vi "gRPC Client Test.vi"(11 "address":string="localhost:") -> (2 "Loop Counter":i32, 3 "Response Data":T1)   [LabVIEW 2019, in "Generated_client.lvlib"]
uses:
  Generated_client.lvlib
  RPC Messages/helloworld_HelloReply.ctl
panel:
  out "Request cluster":cluster{string}
  in  "stop":bool
  out "response error":errorcluster caption="error out"
  out "no error counter":i32
  out "-1014 error counter":i32
  out "-1004 error counter":i32
  out "-1012 error counter 2":i32
  out "destroy error":errorcluster caption="error out"
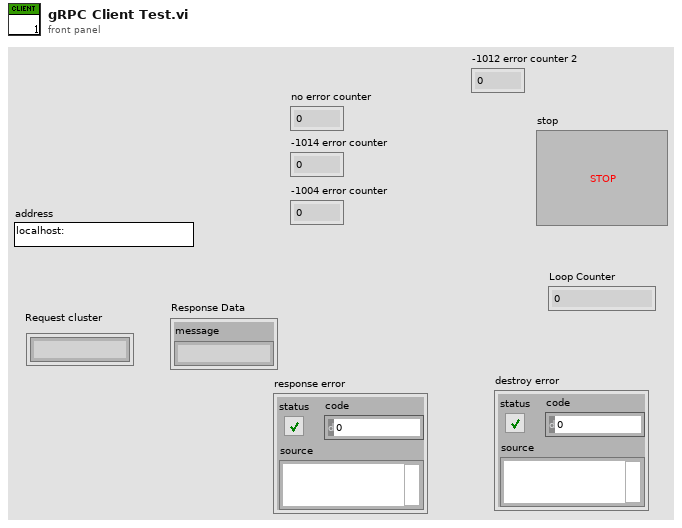
[diagram p1: front panel]
types:
  T1 = typedef "Generated_client.lvlib/helloworld_HelloReply.ctl" = cluster{"message":string}
  T2 = typedef "grpc-lvsupport-release.lvlib/grpcId.ctl" = u64
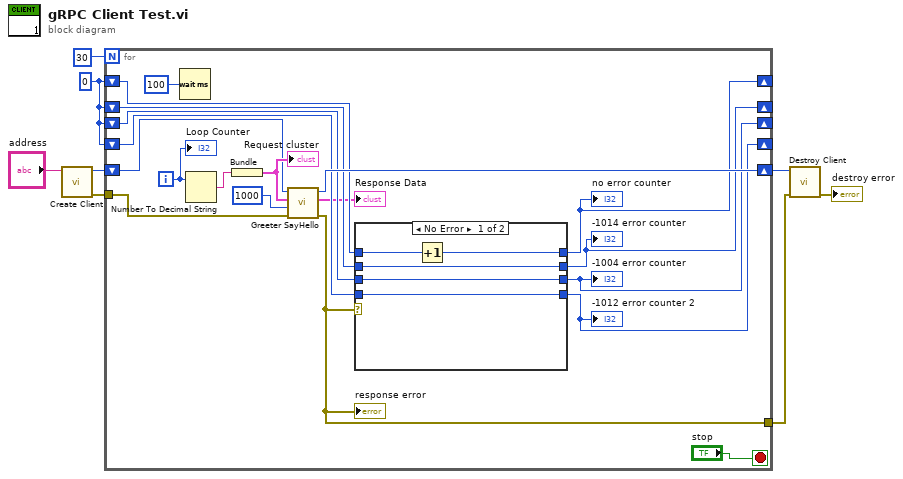
[diagram p0: block diagram]
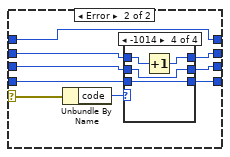
[diagram p2: hidden frame]
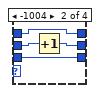
[diagram p4: hidden frame]
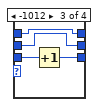
[diagram p5: hidden frame]
diagram:
  w8 = 0
  n1 = call "Create Client.vi"("address"="address") -> ("error out"=w1:errorcluster, "gRPC ID Out"=w6:T2)  [unwired: 9 in]
  n2 = for {
    N: 30 -> [_]
    shift-right: [w27] -> w5
    shift-left: w6 -> [w14]
    shift-right: [w21] -> _
    shift-left: w8 -> [w22]
    shift-right: [w25] -> _
    shift-left: w8 -> [w26]
    shift-right: [w23] -> _
    shift-left: w8 -> [w24]
    shift-right: [w16] -> _
    shift-left: w8 -> [w17]
    tunnel: [w13] -> w3
    tunnel: w1 -> [w10]
    i -> [w20]
    stop <- "stop" stop-if-true
    n3 = Wait (ms)(milliseconds to wait=u32 100) -> ()  [unwired: 1 out]
    n4 = Number To Decimal String(number=w20) -> (decimal integer string=w18:string)  [unwired: 1 in]
    n5 = Bundle(w18) -> (w15:cluster{string})  [unwired: 1 in]
    "Request cluster" <- w15
    n6 = call "Greeter SayHello.vi"("error in"=w10, "timeout (ms)"=1000, "Request Data"=w15, "gRPC ID"=w14) -> ("error out"=w13:errorcluster, "Response Data"=→"Response Data":T1, "gRPC ID out"=w27:T2)  [unwired: 5 in]
    "response error" <- w13
    n7 = case shown="No Error" w13 {
      selector: w13 -> [_ w41]
      tunnel: w26 -> [w30 w39]
      tunnel: [w30 w38] -> w25
      tunnel: w24 -> [w29 w37]
      tunnel: [w29 w36] -> w23
      tunnel: w22 -> [w32 w35]
      tunnel: [w31 w35] -> w21
      tunnel: w17 -> [w28 w34]
      tunnel: [w28 w33] -> w16
      frame No Error {
        n8 = Increment(x=w32) -> (x+1=w31:i32)
      }
      frame Error {
        n9 = Unbundle By Name(w41) -> ("code"=w40:i32)
        n10 = case shown="-1014" w40 {
          tunnel: w39 -> [w44 w46 w49 w56]
          tunnel: [w44 w46 w49 w55] -> w38
          tunnel: w37 -> [w43 w48 w50 w54]
          tunnel: [w43 w47 w50 w54] -> w36
          tunnel: w34 -> [w42 w45 w52 w53]
          tunnel: [w42 w45 w51 w53] -> w33
          frame 0, Default {
          }
          frame -1004 {
            n11 = Increment(x=w48) -> (x+1=w47:i32)
          }
          frame -1012 {
            n12 = Increment(x=w52) -> (x+1=w51:i32)
          }
          frame -1014 {
            n13 = Increment(x=w56) -> (x+1=w55:i32)
          }
        }
      }
    }
    "no error counter" <- w21
    "-1014 error counter" <- w25
    "-1004 error counter" <- w23
    "-1012 error counter 2" <- w16
    "Loop Counter" <- w20
  }
  n14 = call "Destroy Client.vi"("error in"=w3, "gRPC ID"=w5) -> ("error out"=→"destroy error":errorcluster)  [unwired: 9 in]
